vi "Load ROM.vi"(8 "error in (no error)":errorcluster, 11 "EEPROM in":refnum<class "EEPROM.lvclass">) -> (0 "error out":errorcluster, 3 "EEPROM out":refnum<class "EEPROM.lvclass">)   [LabVIEW 2021, in "EEPROM.lvclass"]
uses:
  EEPROM.lvclass
  EEPROM.lvclass/EEPROM.ctl
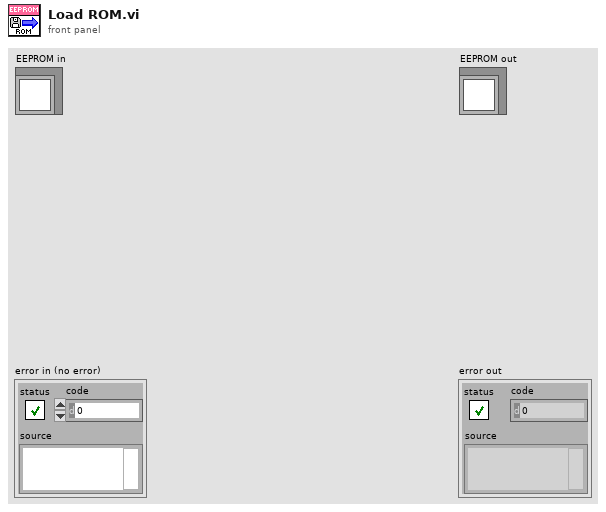
[diagram p1: front panel]
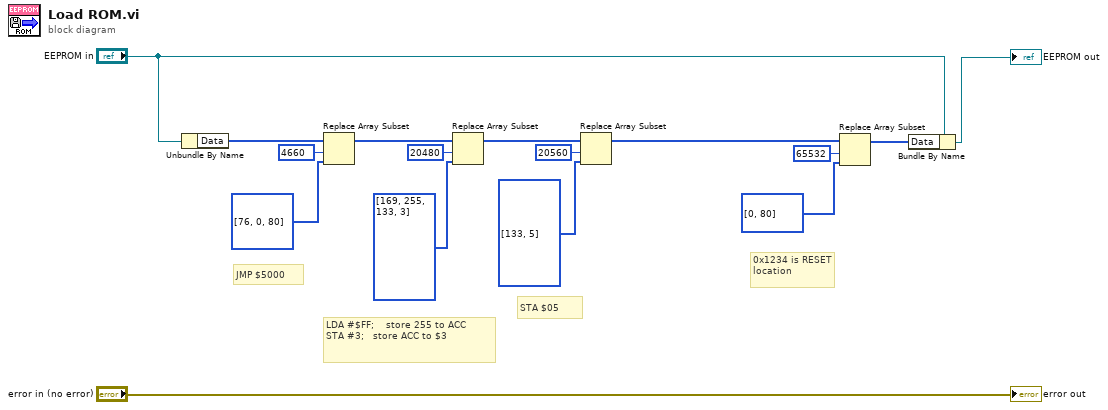
[diagram p0: block diagram]
diagram:
  # "STA $05"
  # "LDA #$FF;    store 255 to ACC\nSTA #3;   store ACC to $3"
  # "0x1234 is RESET location"
  # "JMP $5000"
  n1 = Unbundle By Name("EEPROM in") -> ("Data"=w4:u8[])
  n2 = Replace Array Subset(array=w4, new element=u8[] [76, 0, 80], index=u16 4660) -> (w10:u8[])
  n3 = Replace Array Subset(array=w10, new element=u8[] [169, 255, 133, 3], index=20480) -> (w14:u8[])
  n4 = Replace Array Subset(array=w14, new element=u8[] [133, 5], index=20560) -> (w16:u8[])
  n5 = Replace Array Subset(array=w16, new element=u8[] [0, 80], index=u16 65532) -> (w2:u8[])
  n6 = Bundle By Name(cluster="EEPROM in", "Data"=w2) -> (→"EEPROM out":refnum<class "EEPROM.lvclass">)
  "error out" <- "error in (no error)"
